vi "Process PSD for Preview.vi"(5 "tx config":T1={"rf enable 0"=FALSE, "rf config 0"={"antenna"="TX1", "frequency"=2000000000.0, "lo frequency"=-1.0, "level"=0.0}, "rf enable 1"=FALSE, "rf config 1"={"antenna"="TX1", "frequency"=2000000000.0, "lo frequency"=-1.0, "level"=0.0}, "transfer mode"=enum."Finite", "sample rate"=10000000.0, "start trigger"=enum."Immediate"} {"sample rate" format="%#.3pS/s"; "rf config 0"."level" format="%#_gdBm"; "rf config 0"."lo frequency" format="%#.3pHz"; "rf config 0"."frequency" format="%#.3pHz"; "rf config 1"."level" format="%#_gdBm"; "rf config 1"."lo frequency" format="%#.3pHz"; "rf config 1"."frequency" format="%#.3pHz"}, 6 "Rx?":bool=TRUE, 7 "Rx config":T3={"rf enable 0"=FALSE, "rf config 0"={"antenna"="RX2", "frequency"=2000000000.0, "lo frequency"=-1.0, "level"=0.0}, "rf enable 1"=FALSE, "rf config 1"={"antenna"="RX2", "frequency"=2000000000.0, "lo frequency"=-1.0, "level"=0.0}, "transfer mode"=enum."Finite", "sample rate"=10000000.0, "start trigger"=enum."Immediate"} {"sample rate" format="%#.3pS/s"; "rf config 1"."level" format="%#_gdBm"; "rf config 1"."lo frequency" format="%#.3pHz"; "rf config 1"."frequency" format="%#.3pHz"; "rf config 0"."level" format="%#_gdBm"; "rf config 0"."lo frequency" format="%#.3pHz"; "rf config 0"."frequency" format="%#.3pHz"}, 8 "error in (no error)":errorcluster, 10 "Data Array":u64[](array[numeric])) -> (0 "error out":errorcluster, 3 "Power Spectrum / PSD":cluster{"f0":dbl, "df":dbl, "magnitude":dbl[]})   [LabVIEW 2016]
uses:
  TypeDefs/Rx Config.ctl
  2954/SubVIs/Start Trigger.ctl
  TypeDefs/Tx Config.ctl
  <vilib>/measure/maspectr.llb/FFT Power Spectrum and PSD for 1 Chan (CDB).vi
  <vilib>/measure/NI_MAPro.lvlib
  <instrlib>/_niInstr/DSP/v1/FPGA/niInstr DSP v1 FPGA.lvlib
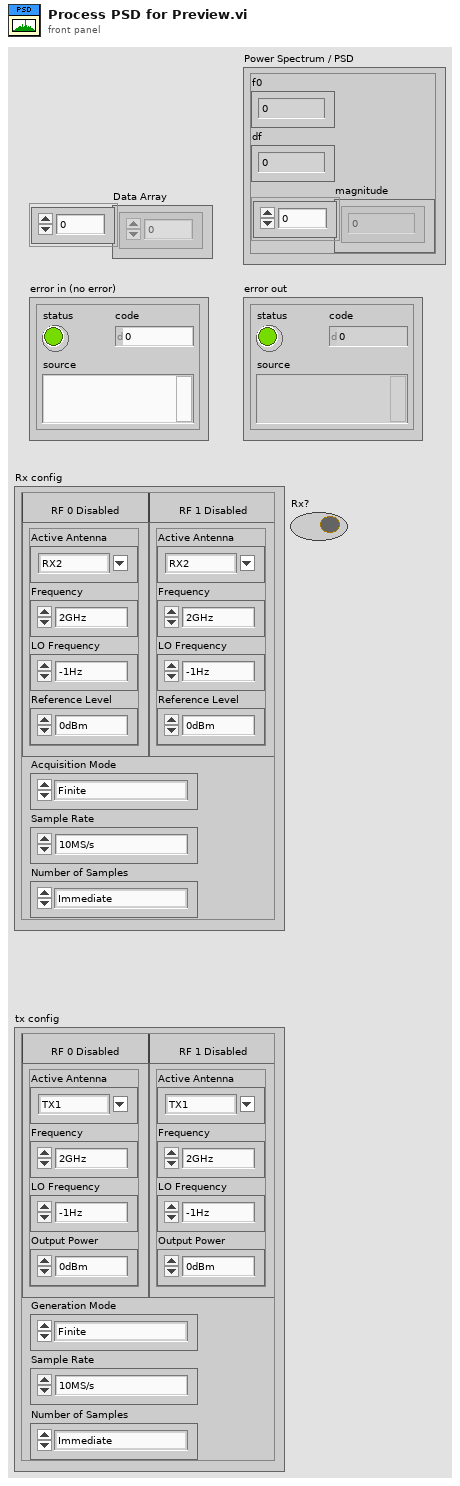
[diagram p1: front panel]
types:
  T1 = typedef "Tx Config.ctl" = cluster{"rf enable 0":bool, "rf config 0":cluster{"antenna":string, "frequency":dbl, "lo frequency":dbl, "level":dbl}, "rf enable 1":bool, "rf config 1":cluster{"antenna":string, "frequency":dbl, "lo frequency":dbl, "level":dbl}, "transfer mode":enum16{"Finite", "Continuous"}, "sample rate":dbl, "start trigger":T2}
  T2 = typedef "Start Trigger.ctl" = enum8{"Software", "Digital Edge", "Rx Start Trigger", "Tx Start Trigger", "Immediate", "Future Time Event"}
  T3 = typedef "Rx Config.ctl" = cluster{"rf enable 0":bool, "rf config 0":cluster{"antenna":string, "frequency":dbl, "lo frequency":dbl, "level":dbl}, "rf enable 1":bool, "rf config 1":cluster{"antenna":string, "frequency":dbl, "lo frequency":dbl, "level":dbl}, "transfer mode":enum16{"Finite", "Continuous"}, "sample rate":dbl, "start trigger":T2}
  T4 = typedef "niInstr DSP v1 Shared.lvlib/IQ Data.ctl" = cluster{"I":fxp<+/-,18,1>, "Q":fxp<+/-,18,1>, "overflow":bool}
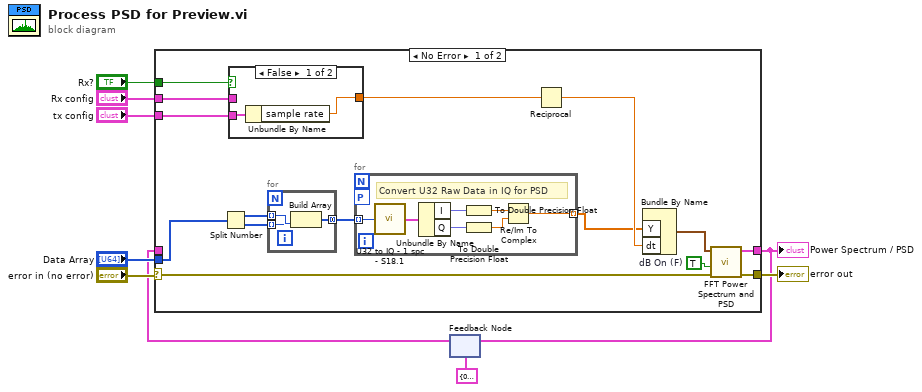
[diagram p0: block diagram]
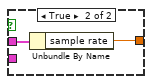
[diagram p2: hidden frame]
diagram:
  n1 = feedback #1(cluster{"f0":dbl, "df":dbl, "magnitude":dbl[]} {"f0"=0.0, "df"=0.0, "magnitude"=[]} ("Power Spectrum / PSD")) -> (w5:cluster{"f0":dbl, "df":dbl, "magnitude":dbl[]})
  n2 = case shown="No Error" "error in (no error)" {
    selector: "error in (no error)" -> [w12 w40]
    tunnel: "Data Array" -> [w13 _]
    tunnel: [w23 w39] -> w6
    tunnel: [w22 w40] -> w8
    tunnel: "Rx config" -> [w20 _]
    tunnel: w5 -> [_ w39]
    tunnel: "Rx?" -> [w19 _]
    tunnel: "tx config" -> [w18 _]
    frame No Error {
      w24 = TRUE  # dB On (F)
      n3 = Split Number(x=w13) -> (hi(x)=w15:u32[], lo(x)=w14:u32[])
      n4 = case shown="False" w19 {
        tunnel: w20 -> [_ w38]
        tunnel: [w35 w37] -> w17
        tunnel: w18 -> [w36 _]
        frame False {
          n5 = Unbundle By Name(w36) -> ("sample rate"=w35:dbl)
        }
        frame True {
          n6 = Unbundle By Name(w38) -> ("sample rate"=w37:dbl)
        }
      }
      n7 = for {
        tunnel: w15 -> [w27] mode=indexing
        tunnel: w14 -> [w26] mode=indexing
        tunnel: [w25] -> w16 mode=concatenating
        n8 = Build Array(w26, w27) -> (w25:u32[])
      }
      n9 = for {
        tunnel: w16 -> [w34] mode=indexing
        tunnel: [w28] -> w11 mode=indexing
        workers-P: _ -> [_]
        # "Convert U32 Raw Data in IQ for PSD"
        n10 = call <instrlib>:"U32 to IQ - 1 spc - S18.1.vi"("U32 data"=w34) -> ("IQ data"=w29:T4)  [unwired: 14 in]
        n11 = Unbundle By Name(w29) -> ("I"=w31:fxp<+/-,18,1>, "Q"=w32:fxp<+/-,18,1>)
        n12 = To Double Precision Float(number=w31) -> (double precision float=w30:dbl)
        n13 = To Double Precision Float(number=w32) -> (double precision float=w33:dbl)
        n14 = Re/Im To Complex(1:w33, 2:w30) -> (0:w28:cdb)
      }
      n15 = Reciprocal(x=w17) -> (1/x=w21:dbl)
      n16 = Bundle By Name("Y"=w11, "dt"=w21) -> (w10:waveform(cdb))  [unwired: 1 in]
      n17 = call-poly <vilib>:"FFT Power Spectrum and PSD.vi"("error in (no error)"=w12, "dB On (F)"=w24, "time signal"=w10) -> ("error out"=w22:errorcluster, "Power Spectrum / PSD"=w23:cluster{"f0":dbl, "df":dbl, "magnitude":dbl[]})  [unwired: 5 in, 2 out]
    }
    frame Error {
    }
  }
  "Power Spectrum / PSD" <- w6
  "error out" <- w8
  n18 = feedback-in #1(w6) -> ()
